vi "Report Unhandled Message ID.vi"(8 "error in (no error)":errorcluster, 11 "Module in":refnum<class "Module.lvclass">) -> (0 "error out":errorcluster, 3 "Module out":refnum<class "Module.lvclass">)   [LabVIEW 2020, in "Volatus.lvlib" / "Module.lvclass"]
uses:
  Module.lvclass
  Module.lvclass/Module.ctl
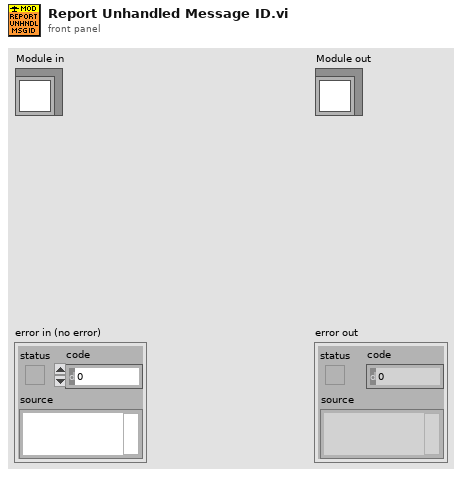
[diagram p1: front panel]
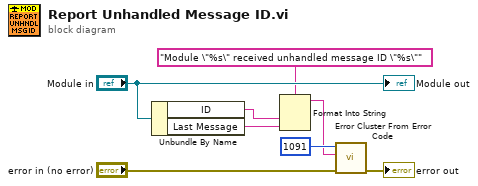
[diagram p0: block diagram]
diagram:
  n1 = Unbundle By Name("Module in") -> ("ID"=w6:string, "Last Message"=w7:string)
  n2 = Format Into String(format string="Module \"%s\" received unhandled message ID \"%s\"", w6, w7) -> (resulting string=w1:string)  [unwired: 2 in, 1 out]
  n3 = call <vilib>:"Error Cluster From Error Code.vi"("error in (no error)"="error in (no error)", "error message (\"\")"=w1, "error code (0)"=1091) -> ("error out"=→"error out":errorcluster)  [unwired: 6 in]
  "Module out" <- "Module in"
